vi "dispose connection.vi"(8 "error in":errorcluster, 11 "connection in":refnum<class "connection.lvclass">) -> (0 "error out":errorcluster)   [LabVIEW 2016, in "connection.lvclass"]
uses:
  connection.lvclass
  connection.lvclass/connection.ctl
  dllwrapper/async tls dl.lvlib
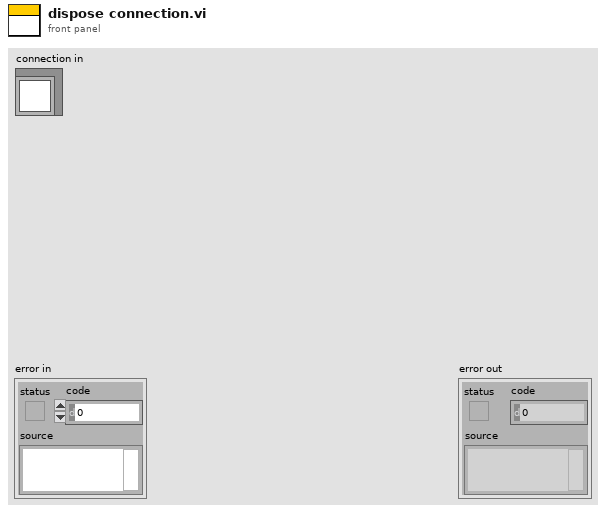
[diagram p1: front panel]
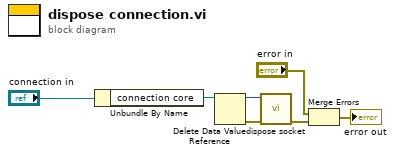
[diagram p0: block diagram]
diagram:
  n1 = Unbundle By Name("connection in") -> ("connection core"=w5:refnum<data-value>)
  n2 = Delete Data Value Reference(data value reference=w5) -> (data value=w3:u64, error out=w2:errorcluster)  [unwired: 1 in]
  n3 = call "dispose socket.vi"("error in"=w2, "socket"=w3) -> ("error out"=w1:errorcluster)  [unwired: 9 in]
  n4 = Merge Errors("error in", w1) -> (→"error out":errorcluster)
